vi "GUI or Akwizycja start.vi"(1 "Akwizycja running?":bool) -> (0 "State":T1)   [LabVIEW 2017]
uses:
  State--enum.ctl
  Application.lvlib
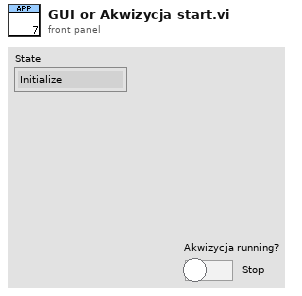
[diagram p1: front panel]
types:
  T1 = typedef "Application.lvlib/State--enum.ctl" = enum16{"Initialize", "Initialize Panel", "UI Interlocks", "Update Status", "Wait for Event", "Exit"}
  T2 = typedef "Application.lvlib/State--enum.ctl" = enum16{"Initialize", "Initialize Panel", "Initialize Panel 2", "UI Interlocks", "Update Status", "Wait for Event", "Akwizycja", "GUI", "Exit"}
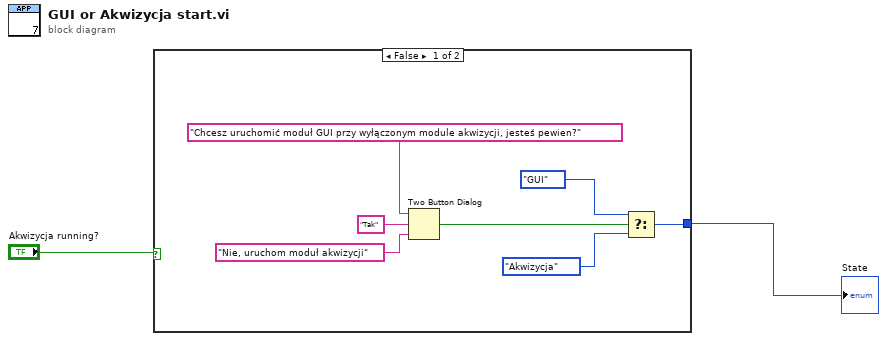
[diagram p0: block diagram]
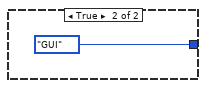
[diagram p2: hidden frame]
diagram:
  n1 = case shown="False" "Akwizycja running?" {
    tunnel: [w3 State--enum."GUI" ("State")] -> w1
    frame False {
      n2 = Two Button Dialog(message="Chcesz uruchomić moduł GUI przy wyłączonym module akwizycji, jesteś pewien?", 1:"Nie, uruchom moduł akwizycji" ("F button name (\"Cancel\")"), 2:"Tak" ("T button name (\"OK\")")) -> (T button?=w8:bool)
      n3 = Select(t=State--enum."GUI" ("State"), s=w8, f=State--enum."Akwizycja" ("State")) -> (s? t:f=w3:T2)
    }
    frame True {
    }
  }
  "State" <- w1
